vi "Memory.vi"(0 "VISA IN":refnum<visa-resource-name>, 5 "error in":errorcluster) -> (14 "VISA Out":refnum<visa-resource-name>, 19 "error out":errorcluster)   [LabVIEW 2018, in "PNA-X.lvlib"]
uses:
  PNA-X.lvlib
panel:
  in  "MathFn":string(combo)="SUBT"
  in  "ON | OFF":bool
  in  "Trace":i32=1
  in  "Window":i32=1
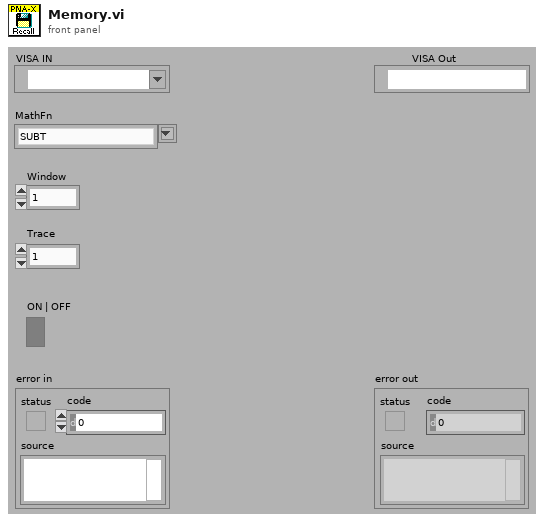
[diagram p1: front panel]
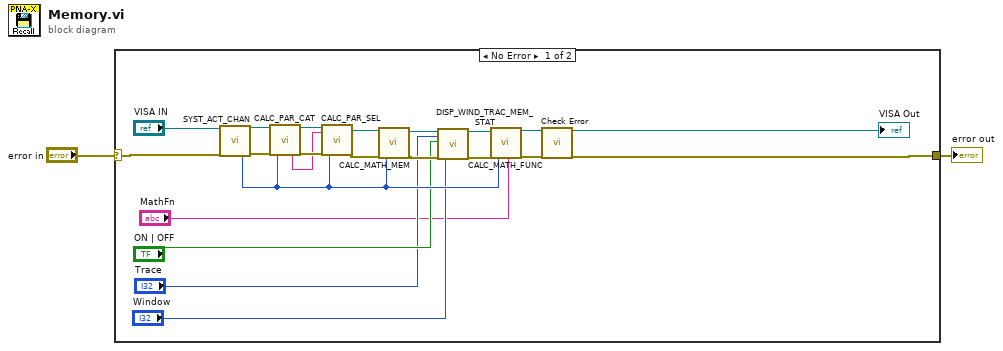
[diagram p0: block diagram]
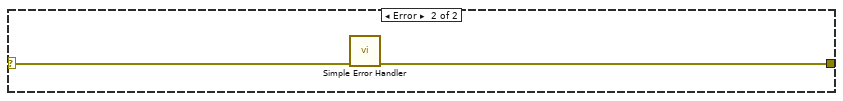
[diagram p2: hidden frame]
diagram:
  n1 = case shown="No Error" "error in" {
    selector: "error in" -> [w19 w26]
    tunnel: [w24 w25] -> w2
    frame No Error {
      n2 = call "SYST_ACT_CHAN.vi"("VISA IN"="VISA IN", "error in"=w19) -> ("Channel"=w13:i32, "VISA Out"=w21:refnum<visa-resource-name>, "error out"=w22:errorcluster)  [unwired: 15 in]
      n3 = call "CALC_PAR_CAT.vi"("VISA IN"=w21, "error in"=w22, "Channel"=w13) -> ("Meas"=w14:string, "VISA Out"=w17:refnum<visa-resource-name>, "error out"=w18:errorcluster)  [unwired: 12 in, 2 out]
      n4 = call "CALC_PAR_SEL.vi"("VISA IN"=w17, "Measurement"=w14, "error in"=w18, "Channel"=w13) -> ("VISA Out"=w16:refnum<visa-resource-name>, "error out"=w15:errorcluster)  [unwired: 14 in]
      n5 = call "CALC_MATH_MEM.vi"("VISA IN"=w16, "error in"=w15, "Channel"=w13) -> ("VISA Out"=w10:refnum<visa-resource-name>, "error out"=w11:errorcluster)  [unwired: 15 in]
      n6 = call "DISP_WIND_TRAC_MEM_STAT.vi"("VISA IN"=w10, "Trace"="Trace", "ON | OFF"="ON | OFF", "error in"=w11, "Window"="Window") -> ("VISA Out"=w7:refnum<visa-resource-name>, "error out"=w6:errorcluster)  [unwired: 13 in]
      n7 = call "CALC_MATH_FUNC.vi"("VISA IN"=w7, "error in"=w6, "Channel"=w13, "Combo Box"="MathFn") -> ("VISA Out"=w4:refnum<visa-resource-name>, "error out"=w5:errorcluster)  [unwired: 14 in]
      n8 = call "Check Error.vi"("VISA Resource Name"=w4, "error in (no error)"=w5) -> ("dup VISA session"=→"VISA Out":refnum<visa-resource-name>, "error out"=w24:errorcluster)  [unwired: 16 in]
    }
    frame Error {
      n9 = call <vilib>:"Simple Error Handler.vi"("error in (no error)"=w26) -> ("error out"=w25:errorcluster)  [unwired: 4 in, 4 out]
    }
  }
  "error out" <- w2
